vi "obtain_stream.vi"(8 "error in (no error)":errorcluster) -> (0 "error out":errorcluster, 3 "log_stream":refnum<queue>)   [LabVIEW 2021, in "system.logging.lvclass"]
uses:
  system.logging.lvclass
  system.logging.lvclass/system.logging.ctl
  severity.ctl
  log_entry.ctl
  service_commands.ctl
  log_stream.ctl
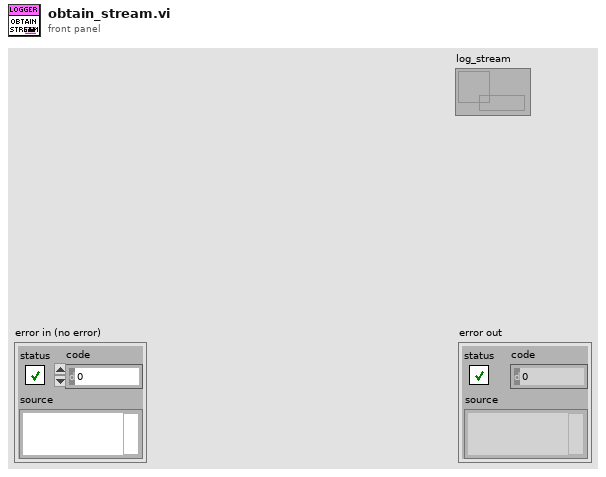
[diagram p1: front panel]
types:
  T1 = typedef "system.logging.lvclass/log_stream.ctl" = cluster{"command":T2, "log_entry":T3}
  T2 = typedef "system.logging.lvclass/service_commands.ctl" = enum16{"close", "log"}
  T3 = typedef "system.logging.lvclass/log_entry.ctl" = cluster{"severity":T4, "message":string, "origin":string, "datetime":timestamp}
  T4 = typedef "system.logging.lvclass/severity.ctl" = enum8{"trace", "debug", "info", "warning", "error"}
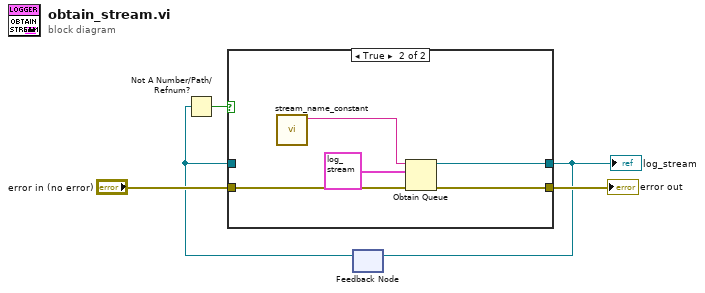
[diagram p0: block diagram]
diagram:
  n1 = feedback #1() -> (w1:refnum<queue>)  [unwired: 1 in]
  n2 = Not A Number/Path/Refnum?(number/path/refnum=w1) -> (NaN/Path/Refnum?=w5:bool)
  n3 = case shown="True" w5 {
    tunnel: "error in (no error)" -> [w7 w11]
    tunnel: [w7 w10] -> w3
    tunnel: [w6 w9] -> w2
    tunnel: w1 -> [w6 _]
    frame False {
    }
    frame True {
      n4 = call "stream_name_constant.vi"() -> ("log_stream_name"=w12:string)  [unwired: 11 in]
      n5 = Obtain Queue(name (unnamed)=w12, element data type=T1 {"command"=enum."close", "log_entry"={"severity"=enum."trace", "message"="", "origin"="", "datetime"=timestamp(0 s since 1904-01-01)}} ("log_stream"), error in (no error)=w11) -> (queue out=w9:refnum<queue>, error out=w10:errorcluster)  [unwired: 2 in, 1 out]
    }
  }
  "error out" <- w3
  "log_stream" <- w2
  n6 = feedback-in #1(w2) -> ()
